vi "Part 2.vi"(11 "Input":string) -> (3 "Output":i64)   [LabVIEW 2021]
uses:
  5450fa51-3a90-40d4-b040-2bae5e58de06.vi
  <userlib>/_OpenG.lib/string/string.llb/Convert EOLs (String)__ogtk.vi
  <vilib>/Comparison/Less/Less Functor/Less Functor.lvclass
panel:
  out "Monkeys":T1(array[cluster])
  in  "Rounds":i32=1000
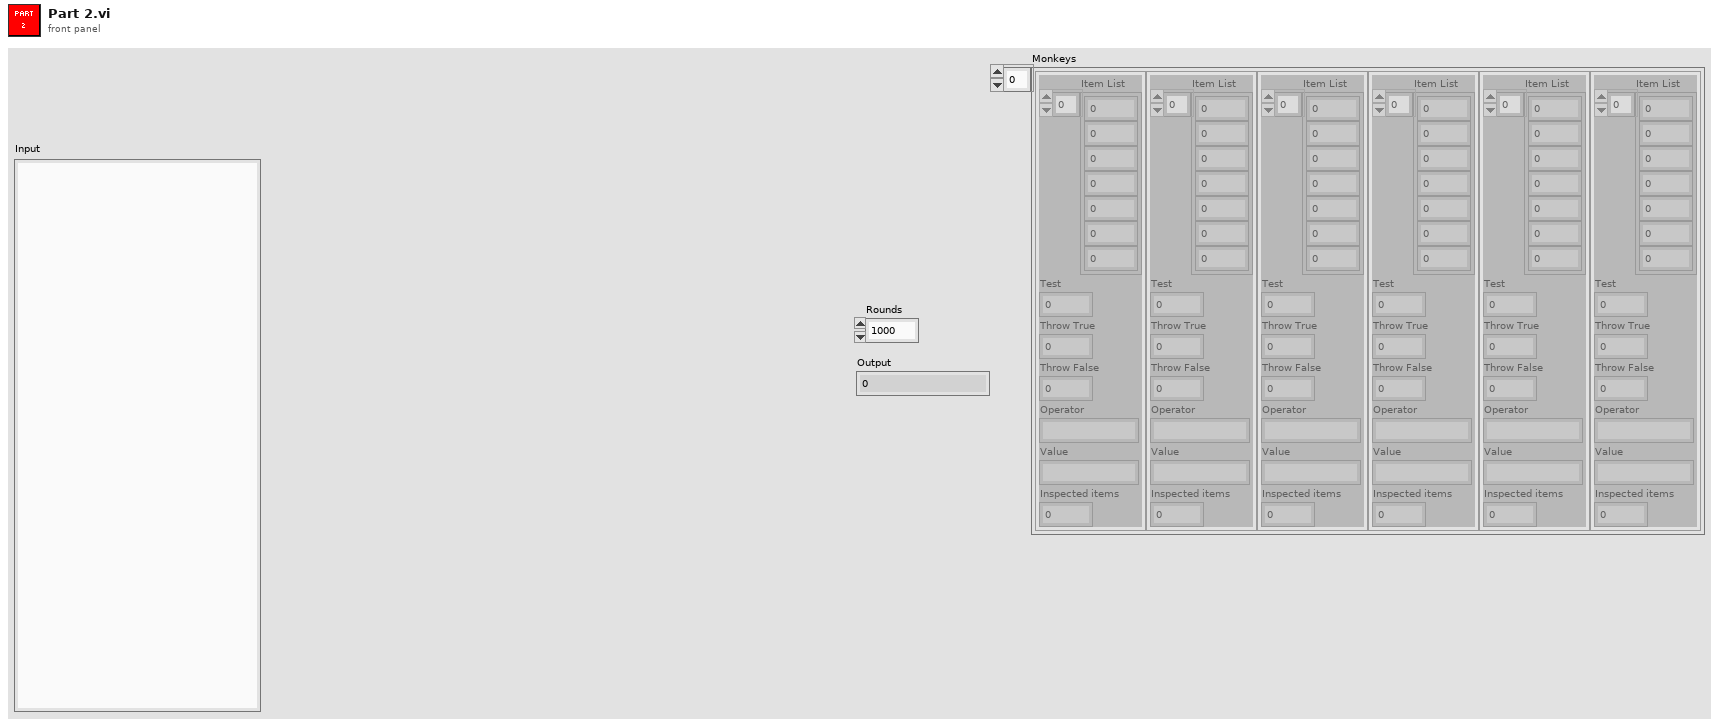
[diagram p1: front panel]
types:
  T1 = cluster{"Item List":u64[], "Test":u64, "Throw True":u64, "Throw False":u64, "Operator":string, "Value":string, "Inspected items":u64}[]
  T2 = cluster{"Item List":u64[], "Test":u64, "Throw True":u64, "Throw False":u64, "Operator":string, "Value":string, "Inspected items":u64}
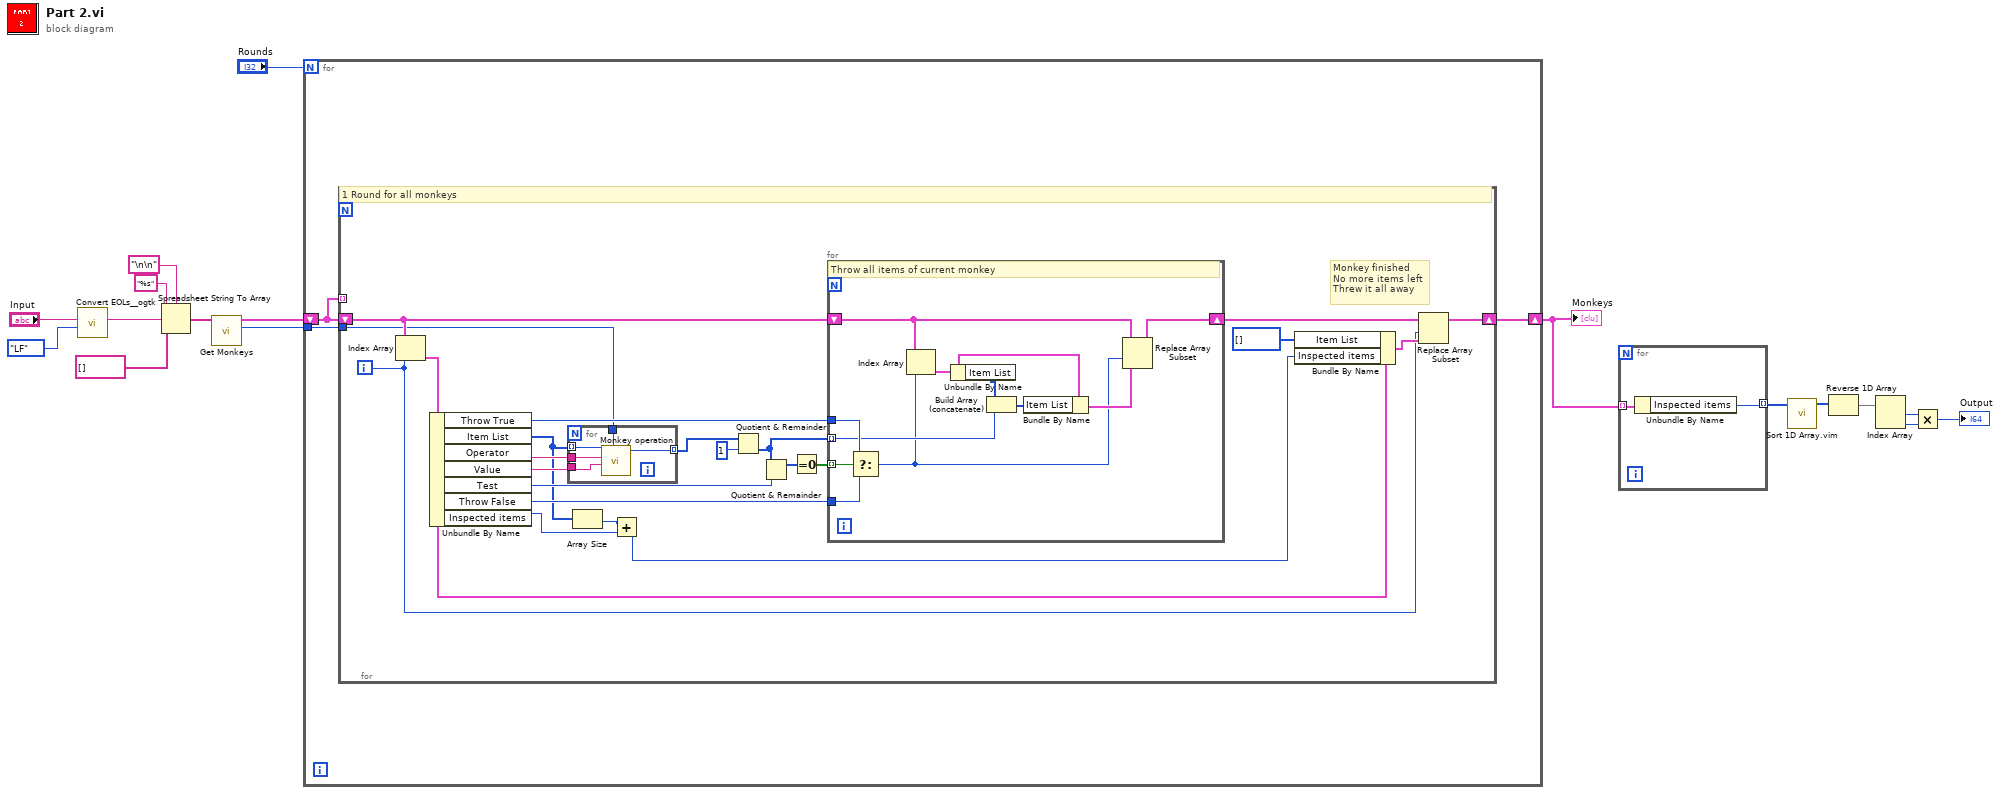
[diagram p0: block diagram]
diagram:
  n1 = call-poly <userlib>:"Convert EOLs__ogtk.vi"("Convert to:"=enum16{"CR", "LF", "CRLF"}."LF", "String in"="Input") -> ("String out"=w16:string)  [unwired: 9 in]
  n2 = Spreadsheet String To Array(delimiter (Tab)="\n\n", format string="%s", spreadsheet string=w16, array type (2D Dbl)=string[] []) -> (array=w14:string[])
  n3 = call "Get Monkeys.vi"("Array in"=w14) -> ("Least Common Multiple"=w2:u64, "Monkeys"=w4:T1)  [unwired: 9 in]
  n4 = for {
    N: "Rounds" -> [_]
    shift-right: [w19] -> w1
    shift-left: w4 -> [w20]
    tunnel: w2 -> [w18]
    n5 = for {
      shift-right: [w41] -> w19
      shift-left: w20 -> [w35]
      tunnel: w20 -> [_] mode=indexing
      tunnel: w18 -> [w21]
      i -> [w32]
      # "Monkey finished\nNo more items left\nThrew it all away"
      # "1 Round for all monkeys"
      n6 = Index Array(array=w35, index=w32) -> (element=w33:T2)
      n7 = Unbundle By Name(w33) -> ("Throw True"=w36:u64, "Item List"=w25:u64[], "Operator"=w28:string, "Value"=w27:string, "Test"=w29:u64, "Throw False"=w30:u64, "Inspected items"=w23:u64)
      n8 = for {
        tunnel: w28 -> [w47]
        tunnel: w27 -> [w46]
        tunnel: w25 -> [w45] mode=indexing
        tunnel: [w44] -> w26 mode=indexing
        tunnel: w21 -> [w43]
        n9 = call "Monkey operation.vi"("Least Common Multiple"=w43, "Value"=w46, "Operator"=w47, "Old"=w45) -> ("New"=w44:u64)  [unwired: 7 in]
      }
      n10 = Array Size(array=w25) -> (size(s)=w24:i32)
      n11 = Add(x=w24, y=w23) -> (x+y=w22:u64)
      n12 = Quotient & Remainder(x=w26, y=u64 1) -> (floor(x/y)=w31:u64[])  [unwired: 1 out]
      n13 = Quotient & Remainder(x=w31, y=w29) -> (x-y*floor(x/y)=w38:u64[])  [unwired: 1 out]
      n14 = Equal To 0?(x=w38) -> (x = 0?=w37:bool[])
      n15 = for {
        tunnel: w37 -> [w58] mode=indexing
        tunnel: w36 -> [w57]
        tunnel: w30 -> [w56]
        shift-right: [w48] -> w34
        shift-left: w35 -> [w49]
        tunnel: w31 -> [w54] mode=indexing
        # "Throw all items of current monkey"
        n16 = Select(t=w57, s=w58, f=w56) -> (s? t:f=w50:u64)
        n17 = Index Array(array=w49, index=w50) -> (element=w53:T2)
        n18 = Unbundle By Name(w53) -> ("Item List"=w55:u64[])
        n19 = Build Array (concatenate)(w55, w54) -> (w52:u64[])
        n20 = Bundle By Name(cluster=w53, "Item List"=w52) -> (w51:T2)
        n21 = Replace Array Subset(array=w49, new element=w51, index=w50) -> (w48:T1)
      }
      n22 = Bundle By Name(cluster=w33, "Item List"=u64[] [], "Inspected items"=w22) -> (w40:T2)
      n23 = Replace Array Subset(array=w34, new element=w40, index=w32) -> (w41:T1)
    }
  }
  "Monkeys" <- w1
  n24 = for {
    tunnel: w1 -> [w60] mode=indexing
    tunnel: [w59] -> w11 mode=indexing
    n25 = Unbundle By Name(w60) -> ("Inspected items"=w59:u64)
  }
  n26 = call "Sort 1D Array.vim"("unsorted array"=w11) -> ("sorted array"=w10:u64[])  [unwired: 10 in]
  n27 = Reverse 1D Array(array=w10) -> (reversed array=w9:u64[])
  n28 = Index Array(array=w9) -> (element #1=w8:u64, element #2=w7:u64)  [unwired: 2 in]
  n29 = Multiply(x=w8, y=w7) -> (x*y=→"Output":u64)
